vi "SetImageData.vi"(8 "error in (no error)":errorcluster, 10 "image data":T1, 11 "Picture in":refnum<class "Image.lvclass">) -> (0 "error out":errorcluster, 3 "Picture out":refnum<class "Image.lvclass">)   [LabVIEW 2021, in "Picture2D.lvlib" / "Image.lvclass"]
uses:
  Image.lvclass
  <vilib>/picture/picture.llb/imagedata.ctl
  Image.lvclass/Image.ctl
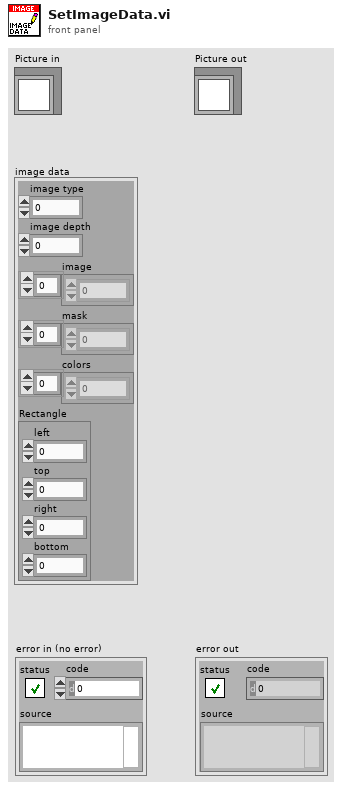
[diagram p1: front panel]
types:
  T1 = typedef "imagedata.ctl" = cluster{"image type":i32, "image depth":i32, "image":u8[], "mask":u8[], "colors":u32[], "Rectangle":cluster{"left":i16, "top":i16, "right":i16, "bottom":i16}}
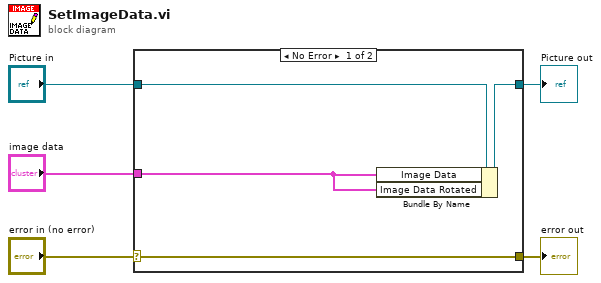
[diagram p0: block diagram]
diagram:
  n1 = case shown="No Error" "error in (no error)" {
    selector: "error in (no error)" -> [w9 w10]
    tunnel: [w9 w10] -> w4
    tunnel: [w7 w11] -> w2
    tunnel: "Picture in" -> [w8 w11]
    tunnel: "image data" -> [w6 _]
    frame No Error {
      n2 = Bundle By Name(cluster=w8, "Image Data"=w6, "Image Data Rotated"=w6) -> (w7:refnum<class "Image.lvclass">)
    }
    frame Error {
    }
  }
  "error out" <- w4
  "Picture out" <- w2
